vi "Merge experiments.vi"(8 "error in (no error)":errorcluster, 10 "Name+Comments+bounds":T1, 11 "Control-Client in":refnum<class "Control-Client.lvclass">) -> (0 "error out":errorcluster, 3 "Control-Client out":refnum<class "Control-Client.lvclass">)   [LabVIEW 2019, in "Control-Client.lvclass"]
uses:
  Control-Client.lvclass
  Experiments/Experiment_merged/Experiment_merged.lvclass
  C:/Users/elysium/Documents/dev/TRANCON/Classes/Experiments/Experiment.lvclass
  Control-Client.lvclass/Control-Client.ctl
  Experiments/Experiment.lvclass/Experiment.ctl
  methods/Read Group #.vi
  Experiments/Experiments_group.lvclass
  Experiments/Experiment.lvclass
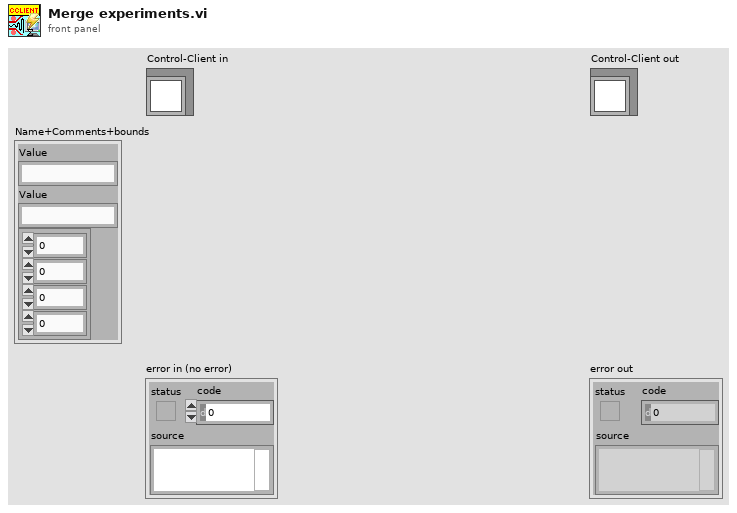
[diagram p1: front panel]
types:
  T1 = cluster{"Value":string, "Value":string, cluster{dbl, dbl, dbl, dbl}}
  T2 = typedef "mylistbox.ctl" = i32[]
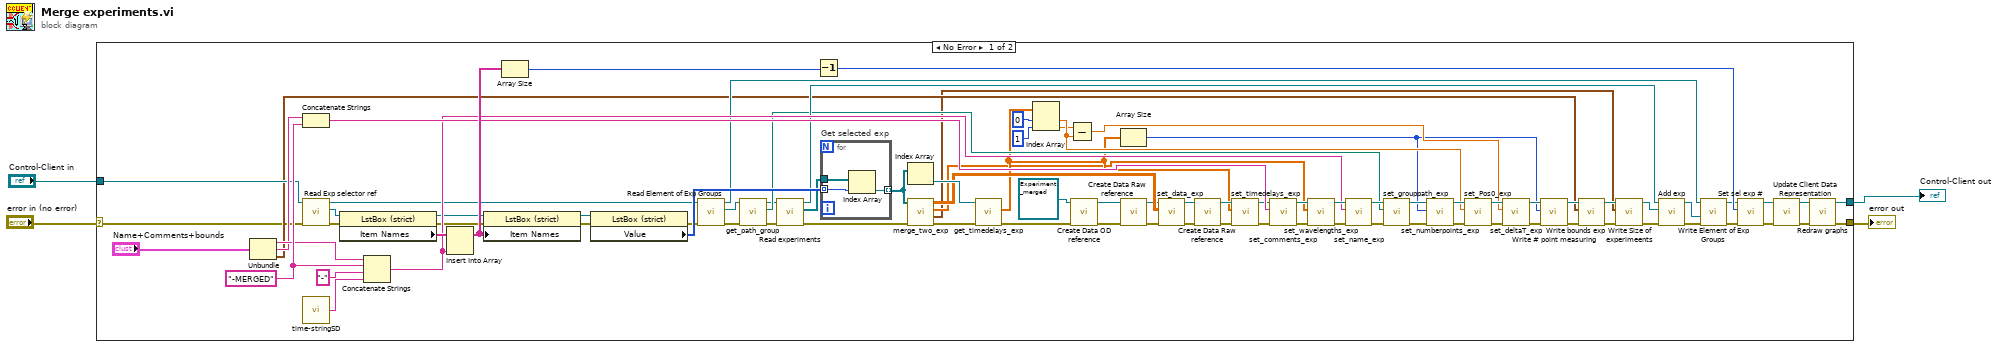
[diagram p0: block diagram]
diagram:
  n1 = case shown="No Error" "error in (no error)" {
    selector: "error in (no error)" -> [w21 w97]
    tunnel: [w55 w97] -> w3
    tunnel: [w54 w96] -> w1
    tunnel: "Control-Client in" -> [w66 w96]
    frame No Error {
      w87 = "-MERGED" ("string")
      n2 = Unbundle("Name+Comments+bounds") -> ("Value"=w86:string, "Value"=w83:string, w28:cluster{dbl, dbl, dbl, dbl})
      n3 = Concatenate Strings(w83, w87) -> (w82:string)
      n4 = call "Read Exp selector ref.vi"("error in (no error)"=w21, "Control-Client in"=w66) -> ("error out"=w71:errorcluster, "Exp selector ref"=w69:refnum<vi>, "Control-Client out"=w22:refnum<class "Control-Client.lvclass">)  [unwired: 7 in]
      n5 = call "time-stringSD.vi"() -> ("time"=w85:string)
      n6 = property on="Property Node" class="LstBox (strict)"(reference=w69, error in=w71) -> (reference out=w15:refnum<vi>, error out=w70:errorcluster, "Item Names"=w92:string[])
      n7 = Concatenate Strings(w86, w87, "-" ("string"), w85) -> (w73:string)
      n8 = Insert Into Array(array=w92, new element=w73) -> (w91:string[])  [unwired: 1 in]
      n9 = property on="Property Node" class="LstBox (strict)"(reference=w15, error in=w70, "Item Names"=w91) -> (reference out=w14:refnum<vi>, error out=w23:errorcluster)
      n10 = Array Size(array=w91) -> (size(s)=w90:i32)
      n11 = property class="LstBox (strict)"(reference=w14, error in=w23) -> (error out=w13:errorcluster, "Value"=w74:T2)  [unwired: 1 out]
      n12 = call "Read Element of Exp Groups.vi"("error in (no error)"=w13, "Control-Client in"=w22) -> ("error out"=w50:errorcluster, "Experiments_group.lvclass"=w47:refnum<class "Experiments_group.lvclass">, "Control-Client out"=w63:refnum<class "Control-Client.lvclass">)  [unwired: 7 in]
      n13 = call "get_path_group.vi"("error in (no error)"=w50, "Experiments_group.lvclass in"=w47) -> ("error out"=w49:errorcluster, "Path"=w48:path, "Experiments_group.lvclass out"=w46:refnum<class "Experiments_group.lvclass">)  [unwired: 7 in]
      n14 = call "Read experiments.vi"("error in (no error)"=w49, "Experiments_group.lvclass in"=w46) -> ("error out"=w67:errorcluster, "Experiments"=w68:refnum<class "Experiment.lvclass">[], "Experiments_group.lvclass out"=w65:refnum<class "Experiments_group.lvclass">)  [unwired: 6 in]
      n15 = Decrement(x=w90) -> (x-1=w72:i32)
      n16 = for "Get selected exp" {
        tunnel: w68 -> [w95]
        tunnel: w74 -> [w94] mode=indexing
        tunnel: [w93] -> w75 mode=indexing
        n17 = Index Array(array=w95, index=w94) -> (element=w93:refnum<class "Experiment.lvclass">)
      }
      n18 = Index Array(array=w75) -> (element=w88:refnum<class "Experiment.lvclass">)  [unwired: 1 in]
      n19 = call "merge_two_exp.vi"("all exp to average"=w75, "error in (no error)"=w67) -> ("averaged without bad points"=w53:dbl[][], "wavelength new"=w11:dbl[], "Array"=w5:cluster{"X pixels":dbl, "Y pixels":dbl}[], "sortie d'erreur"=w89:errorcluster)  [unwired: 5 in]
      n20 = call "get_timedelays_exp.vi"("error in (no error)"=w89, "Experiment.lvclass in"=w88) -> ("error out"=w16:errorcluster, "timedelays"=w12:dbl[])  [unwired: 7 in, 1 out]
      n21 = Index Array(array=w12, index #1=0 ("index"), index #2=1 ("index")) -> (element #1=w36:dbl, element #2=w35:dbl)
      n22 = Subtract(x=w35, y=w36) -> (x-y=w38:dbl)
      n23 = call "Create Data OD reference.vi"("error in (no error)"=w16, "Experiment in"=refnum<class "Experiment_merged.lvclass"> refnum ("Experiment_merged.lvclass")) -> ("error out"=w17:errorcluster, "Experiment out"=w20:refnum<class "Experiment_merged.lvclass">)  [unwired: 8 in]
      n24 = Array Size(array=w12) -> (size(s)=w32:i32)
      n25 = call "Create Data Raw reference.vi"("error in (no error)"=w17, "Experiment in"=w20) -> ("error out"=w18:errorcluster, "Experiment out"=w19:refnum<class "Experiment_merged.lvclass">)  [unwired: 8 in]
      n26 = call "set_data_exp.vi"("error in (no error)"=w18, "Data"=w53, "Experiment.lvclass in"=w19) -> ("error out"=w24:errorcluster, "Experiment.lvclass out"=w27:refnum<class "Experiment_merged.lvclass">)  [unwired: 7 in]
      n27 = call "Create Data Raw reference.vi"("error in (no error)"=w24, "Experiment in"=w27) -> ("error out"=w25:errorcluster, "Experiment out"=w26:refnum<class "Experiment_merged.lvclass">)  [unwired: 8 in]
      n28 = call "set_timedelays_exp.vi"("error in (no error)"=w25, "timedelays"=w12, "Experiment.lvclass in"=w26) -> ("error out"=w79:errorcluster, "Experiment.lvclass out"=w76:refnum<class "Experiment_merged.lvclass">)  [unwired: 7 in]
      n29 = call "set_comments_exp.vi"("error in (no error)"=w79, "Comments"=w82, "Experiment.lvclass in"=w76) -> ("error out"=w80:errorcluster, "Experiment.lvclass out"=w77:refnum<class "Experiment_merged.lvclass">)  [unwired: 7 in]
      n30 = call "set_wavelengths_exp.vi"("error in (no error)"=w80, "wavelengths"=w11, "Experiment.lvclass in"=w77) -> ("error out"=w81:errorcluster, "Experiment.lvclass out"=w78:refnum<class "Experiment_merged.lvclass">)  [unwired: 7 in]
      n31 = call "set_name_exp.vi"("error in (no error)"=w81, "Exp name"=w73, "Experiment.lvclass in"=w78) -> ("error out"=w52:errorcluster, "Experiment.lvclass out"=w51:refnum<class "Experiment_merged.lvclass">)  [unwired: 7 in]
      n32 = call "set_grouppath_exp.vi"("error in (no error)"=w52, "GroupPath"=w48, "Experiment.lvclass in"=w51) -> ("error out"=w42:errorcluster, "Experiment.lvclass out"=w43:refnum<class "Experiment_merged.lvclass">)  [unwired: 7 in]
      n33 = call "set_numberpoints_exp.vi"("error in (no error)"=w42, "numberpoints"=w32, "Experiment.lvclass in"=w43) -> ("error out"=w41:errorcluster, "Experiment.lvclass out"=w45:refnum<class "Experiment_merged.lvclass">)  [unwired: 6 in]
      n34 = call "set_Pos0_exp.vi"("error in (no error)"=w41, "Pos0,ps"=w36, "Experiment.lvclass in"=w45) -> ("error out"=w40:errorcluster, "Experiment.lvclass out"=w44:refnum<class "Experiment_merged.lvclass">)  [unwired: 6 in]
      n35 = call "set_deltaT_exp.vi"("error in (no error)"=w40, "deltaTlast"=w38, "Experiment.lvclass in"=w44) -> ("error out"=w33:errorcluster, "Experiment.lvclass out"=w34:refnum<class "Experiment_merged.lvclass">)  [unwired: 6 in]
      n36 = call "Write # point measuring.vi"("error in (no error)"=w33, "# point measuring"=w32, "Experiment in"=w34) -> ("error out"=w30:errorcluster, "Experiment out"=w29:refnum<class "Experiment_merged.lvclass">)  [unwired: 7 in]
      n37 = call "Write bounds exp.vi"("error in (no error)"=w30, "Bounds"=w28, "Experiment in"=w29) -> ("error out"=w9:errorcluster, "Experiment out"=w8:refnum<class "Experiment_merged.lvclass">)  [unwired: 7 in]
      n38 = call-dynamic "Write Size of experimeents.vi"("error in (no error)"=w9, "Size of experimeents"=w5, "Experiment_merged in"=w8) -> ("error out"=w6:errorcluster, "Experiment_merged out"=w7:refnum<class "Experiment_merged.lvclass">)  [unwired: 7 in]
      n39 = call "Add exp.vi"("error in (no error)"=w6, "New exp"=w7, "Experiments_group in"=w65) -> ("error out"=w60:errorcluster, "Experiments_group out"=w64:refnum<class "Experiments_group.lvclass">)  [unwired: 7 in]
      n40 = call "Write Element of Exp Groups.vi"("error in (no error)"=w60, "Experiments_group.lvclass"=w64, "Control-Client in"=w63) -> ("error out"=w61:errorcluster, "Control-Client out"=w62:refnum<class "Control-Client.lvclass">)  [unwired: 7 in]
      n41 = call "Set sel exp #.vi"("error in (no error)"=w61, "Exp sel #"=w72, "Control-Client in"=w62) -> ("error out"=w58:errorcluster, "Control-Client out"=w59:refnum<class "Control-Client.lvclass">)  [unwired: 7 in]
      n42 = call "Update Client Data Representation.vi"("error in (no error)"=w58, "Control-Client in"=w59) -> ("error out"=w57:errorcluster, "Control-Client out"=w56:refnum<class "Control-Client.lvclass">)  [unwired: 8 in]
      n43 = call "Redraw graphs.vi"("error in (no error)"=w57, "Control-Client in"=w56) -> ("error out"=w55:errorcluster, "Control-Client out"=w54:refnum<class "Control-Client.lvclass">)  [unwired: 8 in]
    }
    frame Error {
    }
  }
  "error out" <- w3
  "Control-Client out" <- w1
